vi "Trial Based Experiment Runner.vi"() -> ()   [LabVIEW 2014]
doc: "Use this template to measure or generate signals using the DAQ Assistant Express VI and NI-DAQmx. Double click the DAQ Assistant Express VI to launch a configuration wizard which steps you through configuring a measurement or generation.\n\nNote: You must have an NI-DAQmx compatible device installed to use this Express VI. Refer to the DAQ Quick Start Guide for NI-DAQ 7.0 for a list of compatible devices."
uses:
  Trial Based Experiment.lvsc/Inputs.ctl
  Trial Based Experiment.lvsc
  Trial Based Experiment.lvsc/Trigger.ctl
  Core SubVIs/Core SubVIs.lvlib
  <vilib>/Statechart/Infrastructure/RTStatechart/RunTime SCN.xnode
  Trial Based Experiment.lvsc/Outputs.ctl
  Trial Based Experiment.lvsc/State.ctl
  Trial Based Experiment.lvsc/StatechartState.ctl
  TrialBasedExperiment.lvclass
  Acquisition/BehaviorData/BehaviorData.lvclass
  <vilib>/Utility/error.llb/DialogType.ctl
  Experiments/ClassDiscrimination/ClassDiscrimination.lvclass
  Experiments/FlePhysEffExperiment/FlePhysEffExperiment.lvclass
  Experiments/MultDimExperiment/MultDimExperiment.lvclass
  Experiments/DotMappingExperiment/DotMappingExperiment.lvclass
  Experiments/EyeCalibration/EyeCalibration.lvclass
  Experiments/FleTraining/FleTraining.lvclass
  Experiments/OriDiscExperiment/OriDiscExperiment.lvclass
  Experiments/WNOriDiscExperiment/WNOriDiscExperiment.lvclass
  Experiments/MoviesExperiment/MoviesExperiment.lvclass
  Experiments/MouseMultiDim/MouseMultiDim.lvclass
  Experiments/MouseBar/MouseBar.lvclass
  Experiments/MouseDotMapping/MouseDotMapping.lvclass
  Experiments/WhiteNoiseOrientationDetection/WhiteNoiseOrientationDetection.lvclass
  <vilib>/Statechart/Common/IntGuid.ctl
  <vilib>/Statechart/Common/NI_SC_LVSCCommonFiles.lvlib
  Trial Based Experiment.lvsc/CompanionDiagram.vi/163/SC Main.vi
  <vilib>/Statechart/Common/DbgID.ctl
  Experiments/CenterSurround/CenterSurround.lvclass
  MatlabExperiment/MatlabExperiment.lvclass
panel:
  out "Stopped 2":bool
  out "Stopped":bool
  in  "Emergency Stop":bool
  out "Data Process Loop":i32
  out "Data Acquire Loop":i32
  out "error out":errorcluster
  out "State":T1
  in  "Experiment":T2(ring)
  out "Missed Updates":dbl
  out "Fixated":bool
  in  "Squirt Time(ms)":u32=50
  in  "Pause":bool
  out "Terminated?":bool
  in  "Stop":bool
  in  "Juice":bool
  # "TODO:\n1. Make EyeParams me properly set\n2. Synchronization"
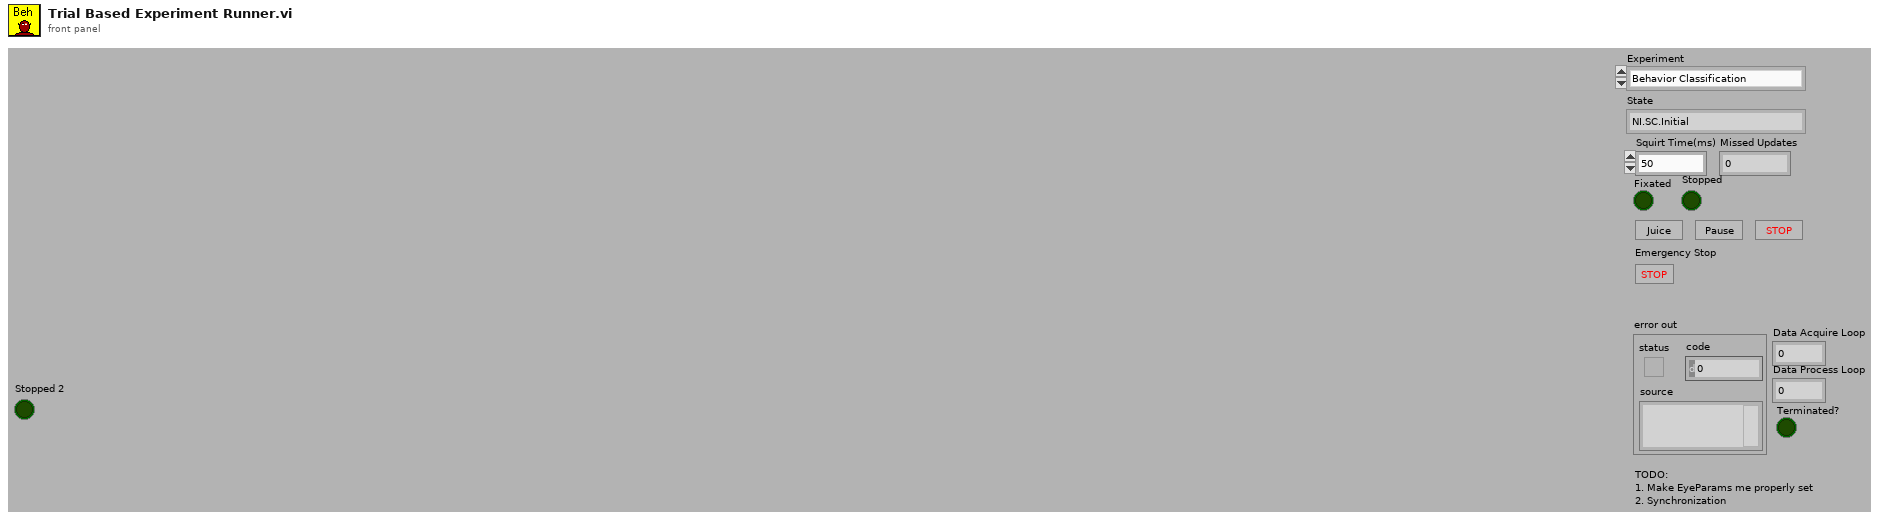
[diagram p1: front panel]
types:
  T1 = typedef "Trial Based Experiment.lvsc/State.ctl" = enum16{"NI.SC.Initial", "NI.SC.History", "NI.SC.ShallowHistory", "NI.SC.Terminal", "Cleanup", "State", "State\\Region\\Pause", "State\\Region\\Response Period", "State\\Region\\Delay Period", "State\\Region\\Hold Fixation", "State\\Region\\Acquire Fixation", "State\\Region\\Abort Trial", "State\\Region\\End Trial", "State\\Region\\Intertrial", "State\\Region\\Start Trial"}
  T2 = enum16{"Behavior Classification", "CenterSurround", "DotMappingExperiment", "Eye Calibration", "FlePhysEffExperiment", "MultDimExperiment", "FlashLagExperiment", "FleTraining", "OriDiscExperiment", "WNOriDetectExperiment", "WNOriDiscExperiment", "MovieExperiment", "MouseMultiDim", "MouseDotMapping", "MouseBarExperiment"}
  T3 = typedef "DialogType.ctl" = u16
  T4 = typedef "StimulationPrimary.ctl" = cluster{"setup":u8, "subject_id":i32, "session_start_time":dbl, "stim_start_time":dbl}
  T5 = typedef "Trial Based Experiment.lvsc/Inputs.ctl" = cluster{"Timing":cluster{"Intertrial time":dbl, "Acquire fixation time":dbl, "Hold fixation time":dbl, "Delay period time":dbl, "Response time":dbl, "Reward":dbl, "Punish time":dbl}, "Stop":bool, "Control states":cluster{"Fixated":bool, "Centered":bool}, "Pause":bool, "Hammer running":bool, "Experiment":refnum<class "TrialBasedExperiment.lvclass">, "error in":errorcluster}
  T6 = typedef "Trial Based Experiment.lvsc/Trigger.ctl" = enum16{"NULL", "Fixated", "Broke Fixation", "Stop", "Correct Response", "Incorrect Response", "Timeout"}
  T7 = enum16{"Get Time", "Get Elapsed Time", "Reset Elapsed Time"}
  T8 = typedef "NI_SC_LVSCCommonFiles.lvlib/IntGuid.ctl" = cluster{"Data1":u32, "Data2":u16, "Data3":u16, "Data4":u8, "Data5":u8, "Data6":u8, "Data11":u8, "Data9":u8, "Data10":u8, "Data8":u8, "Data7":u8}
  T9 = typedef "NI_SC_LVSCCommonFiles.lvlib/DbgID.ctl" = cluster{"VIRef":u32, "IntGUID":T8}
  T10 = typedef "Trial Based Experiment.lvsc/Outputs.ctl" = cluster{"Experiment":refnum<class "TrialBasedExperiment.lvclass">, "Timeout":dbl, "error out":errorcluster}
  T11 = typedef "Trial Based Experiment.lvsc/StatechartState.ctl" = T1[]
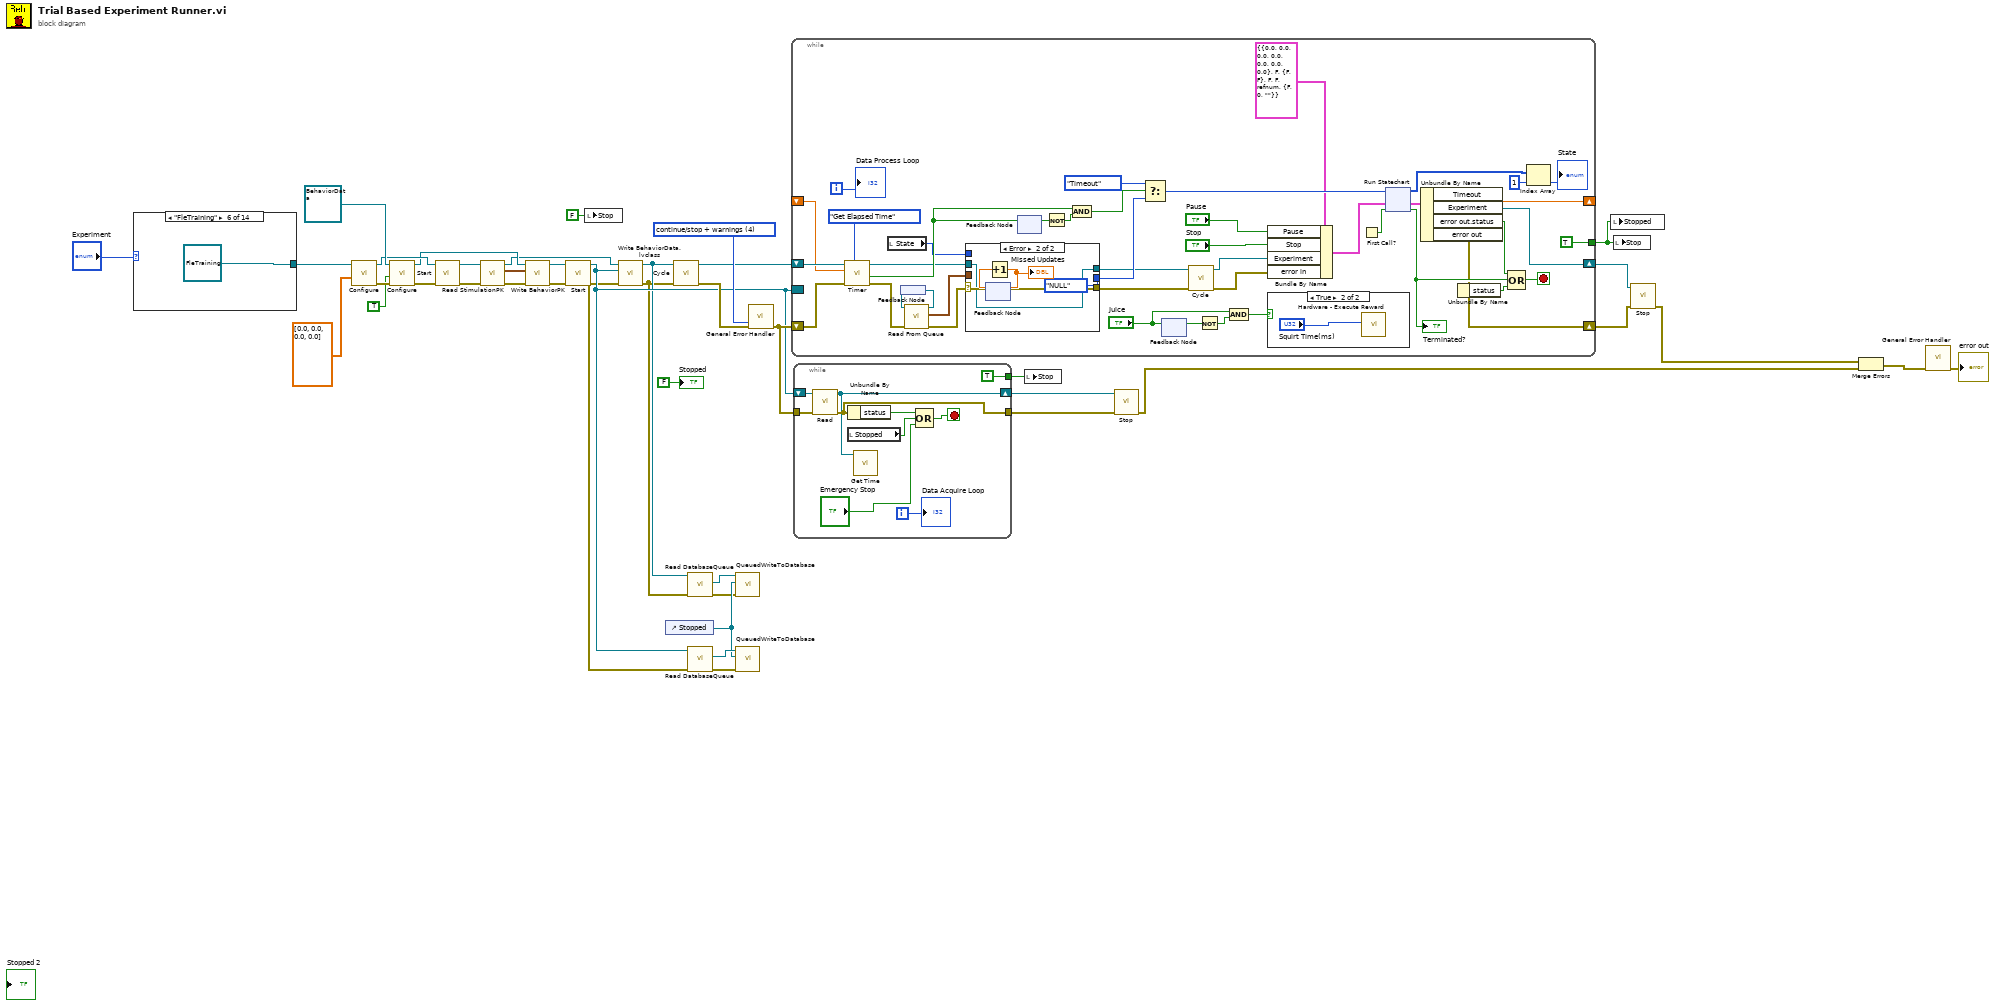
[diagram p0: block diagram]
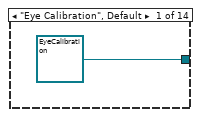
[diagram p2: hidden frame]
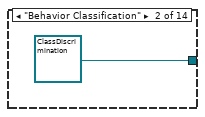
[diagram p3: hidden frame]
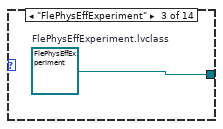
[diagram p4: hidden frame]
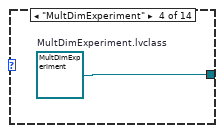
[diagram p5: hidden frame]
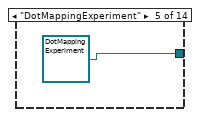
[diagram p6: hidden frame]
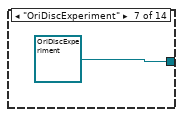
[diagram p7: hidden frame]
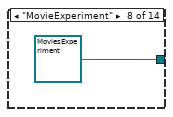
[diagram p8: hidden frame]
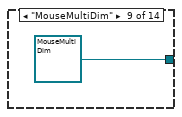
[diagram p9: hidden frame]
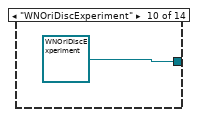
[diagram p10: hidden frame]
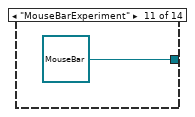
[diagram p11: hidden frame]
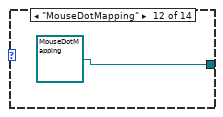
[diagram p12: hidden frame]
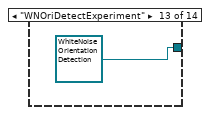
[diagram p13: hidden frame]
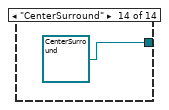
[diagram p14: hidden frame]
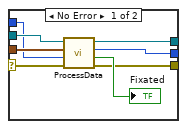
[diagram p15: hidden frame]
diagram:
  w40 = T3 4 items=["no dialog", "OK message", "continue or stop message", "OK message + warnings", "continue/stop + warnings"] ("type of dialog (OK msg:1)")
  n1 = case shown="\"FleTraining\"" "Experiment" {
    tunnel: [refnum<class "EyeCalibration.lvclass"> refnum ("EyeCalibration.lvclass") refnum<class "ClassDiscrimination.lvclass"> refnum ("ClassDiscrimination.lvclass") w44 w45 refnum<class "DotMappingExperiment.lvclass"> refnum ("DotMappingExperiment.lvclass") refnum<class "FleTraining.lvclass"> refnum ("FleTraining.lvclass") refnum<class "OriDiscExperiment.lvclass"> refnum ("OriDiscExperiment.lvclass") refnum<class "MoviesExperiment.lvclass"> refnum ("MoviesExperiment.lvclass") refnum<class "MouseMultiDim.lvclass"> refnum ("MouseMultiDim.lvclass") refnum<class "WNOriDiscExperiment.lvclass"> refnum ("WNOriDiscExperiment.lvclass") refnum<class "MouseBar.lvclass"> refnum ("MouseBar.lvclass") refnum<class "MouseDotMapping.lvclass"> refnum ("MouseDotMapping.lvclass") refnum<class "WhiteNoiseOrientationDetection.lvclass"> refnum ("WhiteNoiseOrientationDetection.lvclass") refnum<class "CenterSurround.lvclass"> refnum ("CenterSurround.lvclass")] -> w34
    frame "Eye Calibration", Default {
    }
    frame "Behavior Classification" {
    }
    frame "FlePhysEffExperiment" {
      w44 = refnum<class "FlePhysEffExperiment.lvclass"> refnum  # FlePhysEffExperiment.lvclass
    }
    frame "MultDimExperiment" {
      w45 = refnum<class "MultDimExperiment.lvclass"> refnum  # MultDimExperiment.lvclass
    }
    frame "DotMappingExperiment" {
    }
    frame "FleTraining" {
    }
    frame "OriDiscExperiment" {
    }
    frame "MovieExperiment" {
    }
    frame "MouseMultiDim" {
    }
    frame "WNOriDiscExperiment" {
    }
    frame "MouseBarExperiment" {
    }
    frame "MouseDotMapping" {
    }
    frame "WNOriDetectExperiment" {
    }
    frame "CenterSurround" {
    }
  }
  n2 = call-dynamic "Configure.vi"("Eye Params"=dbl[] [0.0, 0.0, 0.0, 0.0] ("Init Eye Params"), "TrialBasedExperiment in"=w34) -> ("error out"=w30:errorcluster, "TrialBasedExperiment out"=w29:refnum<class "MatlabExperiment.lvclass">)  [unwired: 8 in]
  n3 = call-dynamic "Configure.vi"("error in (no error)"=w30, "Record"=TRUE, "BehaviorData in"=refnum<class "BehaviorData.lvclass"> refnum ("BehaviorData.lvclass")) -> ("error out"=w24:errorcluster, "BehaviorData out"=w22:refnum<class "BehaviorData.lvclass">)  [unwired: 7 in]
  n4 = call-dynamic "Start.vi"("error in (no error)"=w24, "TrialBasedExperiment in"=w29) -> ("error out"=w25:errorcluster, "TrialBasedExperiment out"=w26:refnum<class "MatlabExperiment.lvclass">)  [unwired: 8 in]
  n5 = call-dynamic "Read StimulationPK.vi"("error in (no error)"=w25, "TrialBasedExperiment in"=w26) -> ("error out"=w19:errorcluster, "StimulationPK"=w23:T4, "TrialBasedExperiment out"=w10:refnum<class "MatlabExperiment.lvclass">)  [unwired: 7 in]
  n6 = call-dynamic "Write BehaviorPK.vi"("error in (no error)"=w19, "BehaviorPK"=w23, "BehaviorData in"=w22) -> ("error out"=w20:errorcluster, "BehaviorData out"=w21:refnum<class "BehaviorData.lvclass">)  [unwired: 7 in]
  n7 = call-dynamic "Start.vi"("error in (no error)"=w20, "Electrophysiology in"=w21) -> ("error out"=w1:errorcluster, "Electrophysiology out"=w7:refnum<class "BehaviorData.lvclass">)  [unwired: 8 in]
  n8 = local write "Stop"(FALSE ("Stop")) -> ()
  n9 = call-dynamic "Write BehaviorData.lvclass.vi"("error in (no error)"=w1, "BehaviorData.lvclass"=w7, "TrialBasedExperiment in"=w10) -> ("error out"=w2:errorcluster, "TrialBasedExperiment out"=w6:refnum<class "MatlabExperiment.lvclass">)  [unwired: 7 in]
  n10 = control-ref of="Stopped"() -> (w4:refnum<vi>)
  n11 = call-dynamic "Cycle.vi"("error in (no error)"=w2, "MatlabExperiment In"=w6) -> ("error out"=w38:errorcluster, "MatlabExperiment Out"=w39:refnum<class "MatlabExperiment.lvclass">)  [unwired: 8 in]
  n12 = call-dynamic "Read DatabaseQueue.vi"("error in (no error)"=w2, "AcquistionObject in"=w6) -> ("error out"=w3:errorcluster, "DatabaseQueue"=w5:refnum<queue>)  [unwired: 7 in, 1 out]
  n13 = call-dynamic "Read DatabaseQueue.vi"("error in (no error)"=w1, "AcquistionObject in"=w7) -> ("error out"=w8:errorcluster, "DatabaseQueue"=w9:refnum<queue>)  [unwired: 7 in, 1 out]
  n14 = call "QueuedWriteToDatabase.vi"("error in"=w3, "Stop Flag Reference"=w4, "queue"=w5) -> ()  [unwired: 8 in, 1 out]
  n15 = call "QueuedWriteToDatabase.vi"("error in"=w8, "Stop Flag Reference"=w4, "queue"=w9) -> ()  [unwired: 8 in, 1 out]
  n16 = call <vilib>:"General Error Handler.vi"("type of dialog (OK msg:1)"=w40, "error in (no error)"=w38) -> ("error out"=w12:errorcluster)  [unwired: 9 in, 4 out]
  n17 = while {
    shift-right: [w89] -> w36
    shift-left: w39 -> [w67]
    shift-right: [w86] -> _
    shift-left: _ -> [w65]
    tunnel: [TRUE] -> w13
    shift-right: [w69] -> w35
    shift-left: w12 -> [w59]
    border: w7 -> [_]
    i -> [w60]
    stop <- w56 stop-if-true
    n18 = call-dynamic "Timer.vi"("Method"=T7."Get Elapsed Time", "error in (no error)"=w59, "Timeout"=w65, "BehaviorData in"=w67) -> ("error out"=w58:errorcluster, "Timeout"=w64:bool, "BehaviorData out"=w61:refnum<class "TrialBasedExperiment.lvclass">)  [unwired: 4 in, 1 out]
    n19 = local read "State"() -> (w57:T1)
    n20 = feedback #1() -> (w62:refnum<class "BehaviorData.lvclass">)
    n21 = call-dynamic "Read From Queue.vi"("error in (no error)"=w58, "BehaviorData in"=w62) -> ("error out"=w72:errorcluster, "Array"=w73:waveform(dbl)[], "BehaviorData out"=w63:refnum<class "BehaviorData.lvclass">)  [unwired: 7 in]
    n22 = feedback-in #1(w63) -> ()
    n23 = case shown="Error" w72 {
      selector: w72 -> [w106 w110]
      tunnel: [w105 w110] -> w70
      tunnel: w73 -> [w104 _]
      tunnel: [w103 Trigger."NULL" ("Trigger")] -> w87
      tunnel: w61 -> [w102 w108]
      tunnel: [w101 w108] -> w71
      tunnel: w57 -> [w100 _]
      frame No Error {
        n24 = call-dynamic "ProcessData.vi"("error in (no error)"=w106, "State"=w100, "Analog Data"=w104, "TrialBasedExperiment in"=w102) -> ("error out"=w105:errorcluster, "Fixated"=→"Fixated":bool, "Trigger"=w103:T6, "TrialBasedExperiment out"=w101:refnum<class "TrialBasedExperiment.lvclass">)  [unwired: 4 in]
      }
      frame Error {
        n25 = feedback #2() -> (w111:dbl)  [unwired: 1 in]
        n26 = Increment(x=w111) -> (x+1=w112:dbl)
        "Missed Updates" <- w112
        n27 = feedback-in #2(w112) -> ()
      }
    }
    n28 = feedback #3() -> (w95:bool)  [unwired: 1 in]
    n29 = feedback-in #3(w64) -> ()
    n30 = Not(x=w95) -> (.not. x?=w94:bool)
    n31 = And(x=w64, y=w94) -> (x .and. y?=w85:bool)
    n32 = Select(t=Trigger."Timeout" ("Trigger"), s=w85, f=w87) -> (s? t:f=w80:T6)
    n33 = feedback #4() -> (w93:bool)  [unwired: 1 in]
    n34 = feedback-in #4("Juice") -> ()
    n35 = call-dynamic "Cycle.vi"("error in (no error)"=w70, "TrialBasedExperiment In"=w71) -> ("error out"=w81:errorcluster, "TrialBasedExperiment Out"=w84:refnum<class "TrialBasedExperiment.lvclass">)  [unwired: 8 in]
    n36 = Not(x=w93) -> (.not. x?=w92:bool)
    n37 = And(x="Juice", y=w92) -> (x .and. y?=w90:bool)
    n38 = case shown="True" w90 {
      frame False {
      }
      frame True {
        n39 = call "Hardware - Execute Reward.vi"("Reward Time (200 ms)"="Squirt Time(ms)") -> ()  [unwired: 1 in, 10 out]
      }
    }
    n40 = Bundle By Name(cluster=T5 {"Timing"={"Intertrial time"=0.0, "Acquire fixation time"=0.0, "Hold fixation time"=0.0, "Delay period time"=0.0, "Response time"=0.0, "Reward"=0.0, "Punish time"=0.0}, "Stop"=FALSE, "Control states"={"Fixated"=FALSE, "Centered"=FALSE}, "Pause"=FALSE, "Hammer running"=FALSE, "Experiment"=refnum, "error in"={"status"=FALSE, "code"=0, "source"=""}} ("Inputs"), "Pause"="Pause", "Stop"="Stop", "Experiment"=w84, "error in"=w81) -> (w79:T5)
    n41 = First Call?() -> (First Call?: T/F=w97:bool)
    n42 = xnode "Run Statechart"("Init?"=w97, "Inputs"=w79, "Trigger"=w80) -> ("Terminated?"=w82:bool, "Outputs"=w96:T10, "Active States"=w78:T11)
    "Terminated?" <- w82
    n43 = Unbundle By Name(w96) -> ("Timeout"=w86:dbl, "Experiment"=w89:refnum<class "TrialBasedExperiment.lvclass">, "error out.status"=w83:bool, "error out"=w69:errorcluster)
    n44 = Unbundle By Name(w69) -> ("status"=w68:bool)
    n45 = Compound Arithmetic op=OR(w83, w82, w68) -> (w56:bool)
    n46 = Index Array(array=w78, index=1) -> (element=→"State":T1)
    "Data Process Loop" <- w60
  }
  n47 = while {
    tunnel: [w210] -> w18
    tunnel: w12 -> [w209]
    shift-right: [w206] -> w17
    shift-left: w7 -> [w213]
    tunnel: [TRUE] -> w33
    i -> [w208]
    stop <- w211 stop-if-true
    n48 = call-dynamic "Read.vi"("error in (no error)"=w209, "Behavior in"=w213) -> ("error out"=w210:errorcluster, "Behavior out"=w206:refnum<class "BehaviorData.lvclass">)  [unwired: 8 in]
    n49 = local read "Stopped"() -> (w204:bool)
    n50 = Unbundle By Name(w210) -> ("status"=w212:bool)
    n51 = call-dynamic "Get Time.vi"("BehaviorData in"=w206) -> ()  [unwired: 8 in, 3 out]
    n52 = Compound Arithmetic op=OR(w212, w204, "Emergency Stop") -> (w211:bool)
    "Data Acquire Loop" <- w208
  }
  n53 = local write "Stop"(w33) -> ()
  n54 = call-dynamic "Stop.vi"("error in (no error)"=w18, "Electrophysiology in"=w17) -> ("error out"=w16:errorcluster)  [unwired: 8 in, 1 out]
  n55 = local write "Stopped"(w13) -> ()
  n56 = local write "Stop"(w13) -> ()
  n57 = call-dynamic "Stop.vi"("error in (no error)"=w35, "TrialBasedExperiment in"=w36) -> ("error out"=w15:errorcluster)  [unwired: 8 in, 1 out]
  n58 = Merge Errors(w15, w16) -> (w11:errorcluster)
  n59 = call <vilib>:"General Error Handler.vi"("error in (no error)"=w11) -> ("error out"=→"error out":errorcluster)  [unwired: 10 in, 4 out]
  "Stopped" <- FALSE ("Stopped")
